vi "TEST_DATA_1.vi"() -> ()   [LabVIEW 2021]
panel:
  out "Numeric":dbl
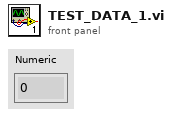
[diagram p1: front panel]
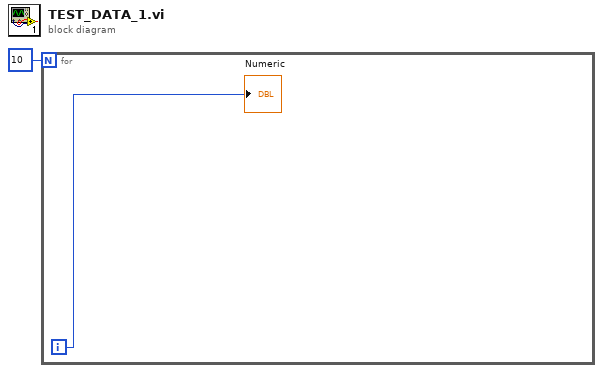
[diagram p0: block diagram]
diagram:
  n1 = for {
    N: 10 -> [_]
    i -> [w2]
    "Numeric" <- w2
  }
